vi "Add(I64).vi"(1 "Enable(T)":bool=TRUE, 2 "In":i64, 4 "n":i64=1) -> (6 "Out":i64=1)   [LabVIEW 2013]
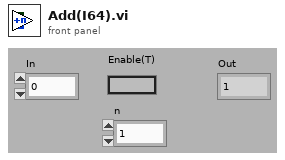
[diagram p1: front panel]
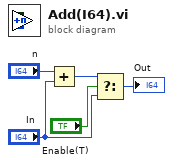
[diagram p0: block diagram]
diagram:
  n1 = Add(x="n", y="In") -> (x+y=w1:i64)
  n2 = Select(t=w1, s="Enable(T)", f="In") -> (s? t:f=→"Out":i64)
